vi "1D Average.vi"(11 "1D array":dbl[](array[numeric])) -> (3 "average value":dbl)   [LabVIEW 2013]
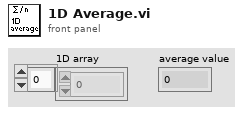
[diagram p1: front panel]
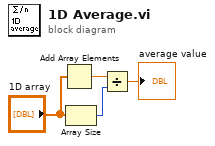
[diagram p0: block diagram]
diagram:
  n1 = Add Array Elements(numeric array="1D array") -> (sum=w3:dbl)
  n2 = Array Size(array="1D array") -> (size(s)=w1:i32)
  n3 = Divide(x=w3, y=w1) -> (x/y=→"average value":dbl)
